vi "Read_diagnosis_data.vi"(11 "configuration file path":path) -> (2 "acelerometros":dbl, 3 "WD":dbl)   [LabVIEW 2015]
uses:
  <vilib>/Utility/config.llb/Read Key (Double).vi
  <vilib>/Utility/config.llb/NI_LVConfig.lvlib
panel:
  out "error out":errorcluster
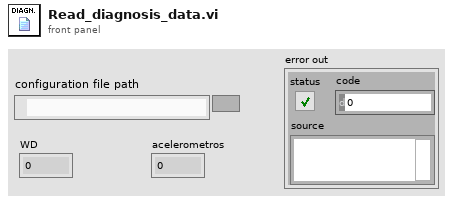
[diagram p1: front panel]
types:
  T1 = typedef "NI_LVConfig.lvlib/Config Data RefNum.ctl" = refnum<k1>
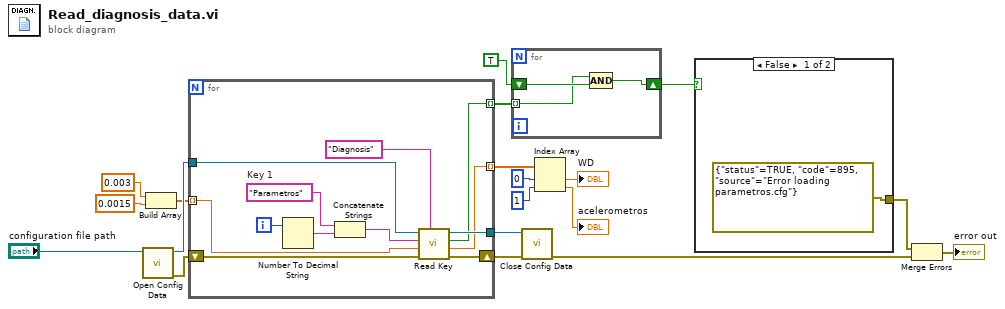
[diagram p0: block diagram]
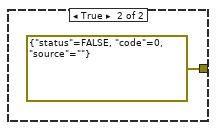
[diagram p2: hidden frame]
diagram:
  n1 = call <vilib>:"Open Config Data.vi"("configuration file path"="configuration file path") -> ("error out"=w18:errorcluster, "refnum"=w19:T1)  [unwired: 2 in, 7 out]
  n2 = Build Array(0.003 ("element"), 0.0015 ("element")) -> (w11:dbl[])
  n3 = for {
    tunnel: w19 -> [w26]
    shift-right: [w24] -> w3
    shift-left: w18 -> [w25]
    tunnel: [w23] -> w4
    tunnel: [w20] -> w14 mode=indexing
    tunnel: w11 -> [w22] mode=indexing
    tunnel: [w21] -> w10 mode=indexing
    i -> [w30]
    w28 = "Parametros"  # Key 1
    n4 = Number To Decimal String(number=w30) -> (decimal integer string=w29:string)  [unwired: 1 in]
    n5 = Concatenate Strings(w28, w29) -> (w27:string)
    n6 = call-poly <vilib>:"Read Key.vi"("section"="Diagnosis", "error in (no error)"=w25, "default value"=w22, "key"=w27, "refnum"=w26) -> ("error out"=w24:errorcluster, "value"=w21:dbl, "found?"=w20:bool, "refnum out"=w23:T1)  [unwired: 3 in]
  }
  n7 = for {
    shift-right: [w33] -> w15
    shift-left: TRUE -> [w34]
    tunnel: w14 -> [w32] mode=indexing
    n8 = Compound Arithmetic op=AND(w32, w34) -> (w33:bool)
  }
  n9 = call <vilib>:"Close Config Data.vi"("error in (no error)"=w3, "refnum"=w4) -> ("error out"=w5:errorcluster)  [unwired: 8 in, 1 out]
  n10 = Index Array(array=w10, index #1=0 ("index"), index #2=1 ("index")) -> (element #1=→"WD":dbl, element #2=→"acelerometros":dbl)
  n11 = case shown="False" w15 {
    tunnel: [errorcluster {"status"=TRUE, "code"=895, "source"="Error loading parametros.cfg"} ("error out") errorcluster {"status"=FALSE, "code"=0, "source"=""} ("error out")] -> w2
    frame False {
    }
    frame True {
    }
  }
  n12 = Merge Errors(w2, w5) -> (→"error out":errorcluster)
